vi "Producción_VAR_LOCALES.vi"() -> ()   [LabVIEW 2021]
panel:
  out "Meter":i32(knob) scale=0.0..10.0
  out "Iteraciones de consumo":i32
  in  "Tiempo de consumo":u32=10
  out "Gráfica de consumo":dbl(graph)
  out "Grafica de produccion":dbl(graph)
  in  "Tiempo de produccion":u32=10
  in  "Stop":bool
  out "Iteraciones de produccion":i32
  # "Mendoza Meza Manuel Everardo"
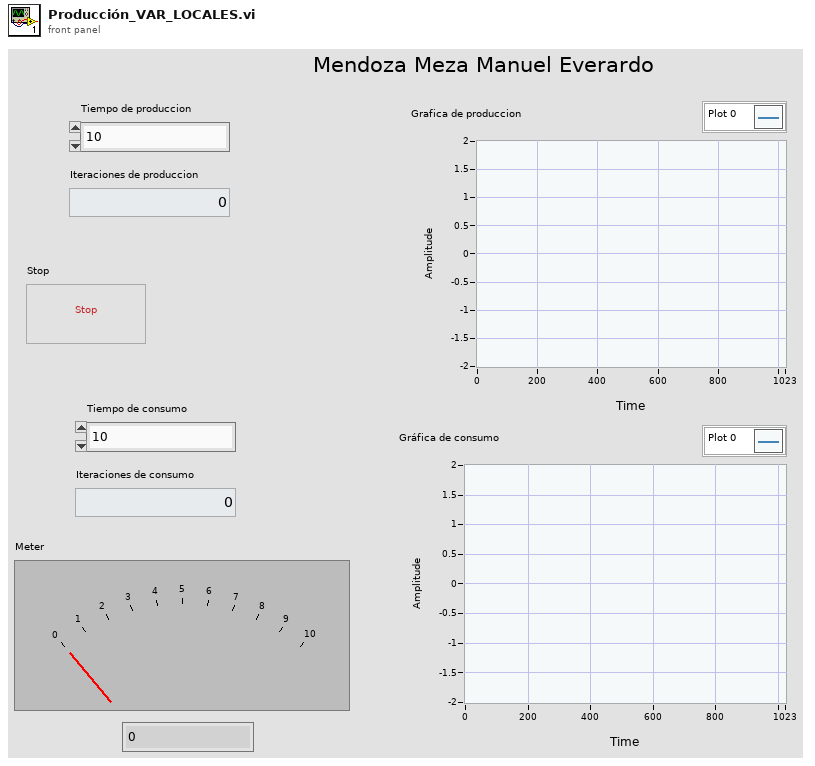
[diagram p1: front panel]
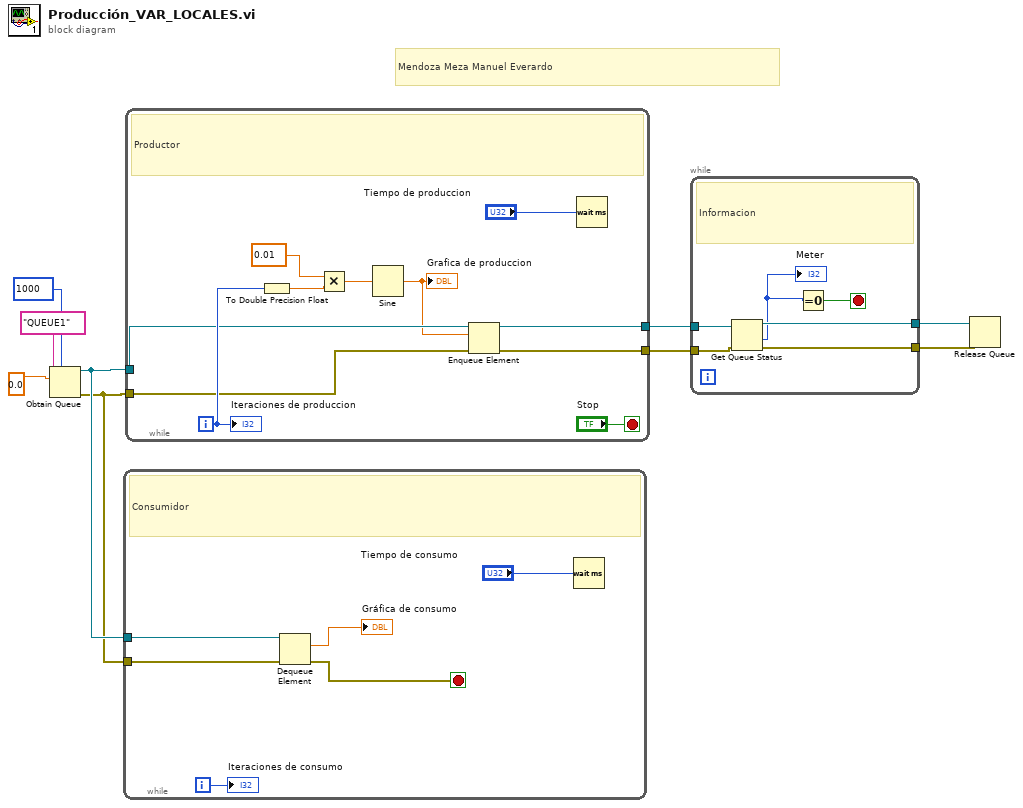
[diagram p0: block diagram]
diagram:
  # "Mendoza Meza Manuel Everardo"
  n1 = Obtain Queue(max queue size (-1, unlimited)=1000, name (unnamed)="QUEUE1", element data type=0.0) -> (queue out=w6:refnum<queue>, error out=w5:errorcluster)  [unwired: 2 in, 1 out]
  n2 = while {
    tunnel: w6 -> [w13]
    tunnel: w5 -> [w12]
    i -> [w14]
    stop <- w10 stop-if-true
    # "Consumidor"
    n3 = Dequeue Element(queue=w13, error in (no error)=w12) -> (element=→"Gráfica de consumo":dbl, error out=w10:errorcluster)  [unwired: 1 in, 2 out]
    n4 = Wait (ms)(milliseconds to wait="Tiempo de consumo") -> ()  [unwired: 1 out]
    "Iteraciones de consumo" <- w14
  }
  n5 = while {
    tunnel: w6 -> [w20]
    tunnel: w5 -> [w19]
    tunnel: [w17] -> w3
    tunnel: [w16] -> w4
    i -> [w24]
    stop <- "Stop" stop-if-true
    # "Productor"
    n6 = To Double Precision Float(number=w24) -> (double precision float=w22:dbl)
    n7 = Multiply(x=0.01, y=w22) -> (x*y=w21:dbl)
    n8 = Sine(x=w21) -> (sin(x)=w18:dbl)
    "Grafica de produccion" <- w18
    n9 = Enqueue Element(queue=w20, element=w18, error in (no error)=w19) -> (queue out=w17:refnum<queue>, error out=w16:errorcluster)  [unwired: 1 in, 1 out]
    n10 = Wait (ms)(milliseconds to wait="Tiempo de produccion") -> ()  [unwired: 1 out]
    "Iteraciones de produccion" <- w24
  }
  n11 = while {
    tunnel: w4 -> [w32]
    tunnel: w3 -> [w31]
    tunnel: [w30] -> w2
    tunnel: [w29] -> w1
    stop <- w28 stop-if-true
    # "Informacion"
    n12 = Get Queue Status(queue=w31, error in (no error)=w32) -> (queue out=w29:refnum<queue>, # pending insert=w27:i32, error out=w30:errorcluster)  [unwired: 1 in, 5 out]
    "Meter" <- w27
    n13 = Equal To 0?(x=w27) -> (x = 0?=w28:bool)
  }
  n14 = Release Queue(queue=w1, error in (no error)=w2) -> ()  [unwired: 1 in, 3 out]
